vi "Heure en secondes.vi"() -> (0 "Heure en milisecondes":u32, 1 "Heure en secondes":u32)   [LabVIEW 2020, in "Library Commun.lvlib"]
uses:
  Library Commun.lvlib
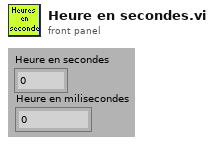
[diagram p1: front panel]
types:
  T1 = typedef "LVDateTimeRec.ctl" = cluster{"fraction de seconde":dbl, "seconde":i32, "minute":i32, "heure":i32, "jour du mois":i32, "mois":i32, "année":i32, "jour de la semaine":i32, "jour de l'année":i32, "DST":i32}
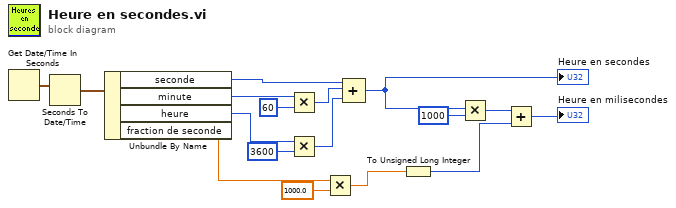
[diagram p0: block diagram]
diagram:
  n1 = Get Date/Time In Seconds() -> (seconds since 1Jan1904=w17:timestamp)
  n2 = Seconds To Date/Time(time stamp (now)=w17) -> (date time rec=w16:T1)  [unwired: 1 in]
  n3 = Unbundle By Name(w16) -> ("seconde"=w11:i32, "minute"=w15:i32, "heure"=w12:i32, "fraction de seconde"=w7:dbl)
  n4 = Multiply(x=w15, y=60) -> (x*y=w10:i32)
  n5 = Multiply(x=w12, y=3600) -> (x*y=w9:i32)
  n6 = Multiply(x=w7, y=1000.0) -> (x*y=w3:dbl)
  n7 = Compound Arithmetic op=ADD(w11, w10, w9) -> (w6:i32)
  "Heure en secondes" <- w6
  n8 = To Unsigned Long Integer(number=w3) -> (unsigned 32bit integer=w2:u32)
  n9 = Multiply(x=w6, y=1000) -> (x*y=w4:i32)
  n10 = Add(x=w4, y=w2) -> (x+y=→"Heure en milisecondes":u32)
